vi "gfitsio-error-cluster-from-code.vi"(8 "error in (no error)":errorcluster, 11 "error code":i32) -> (0 "error out":errorcluster)   [LabVIEW 2019, in "gfitsio.lvlib"]
doc: "Converts an error code to an error cluster. If the CFITSIO error stack contains messages, these are placed in the \"source\" field of <B>error out</B>. If <B>error in</B> indicates that an error occurred before this VI or function ran, <B>error out</B> contains the same error information. Otherwise, it describes the error status corresponding to the <B>error code</B>."
uses:
  gfitsio.lvlib
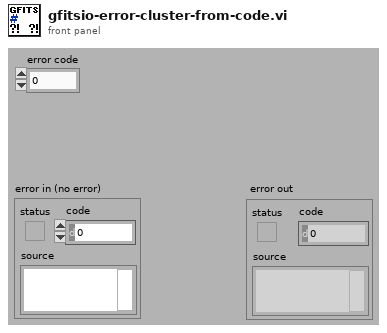
[diagram p1: front panel]
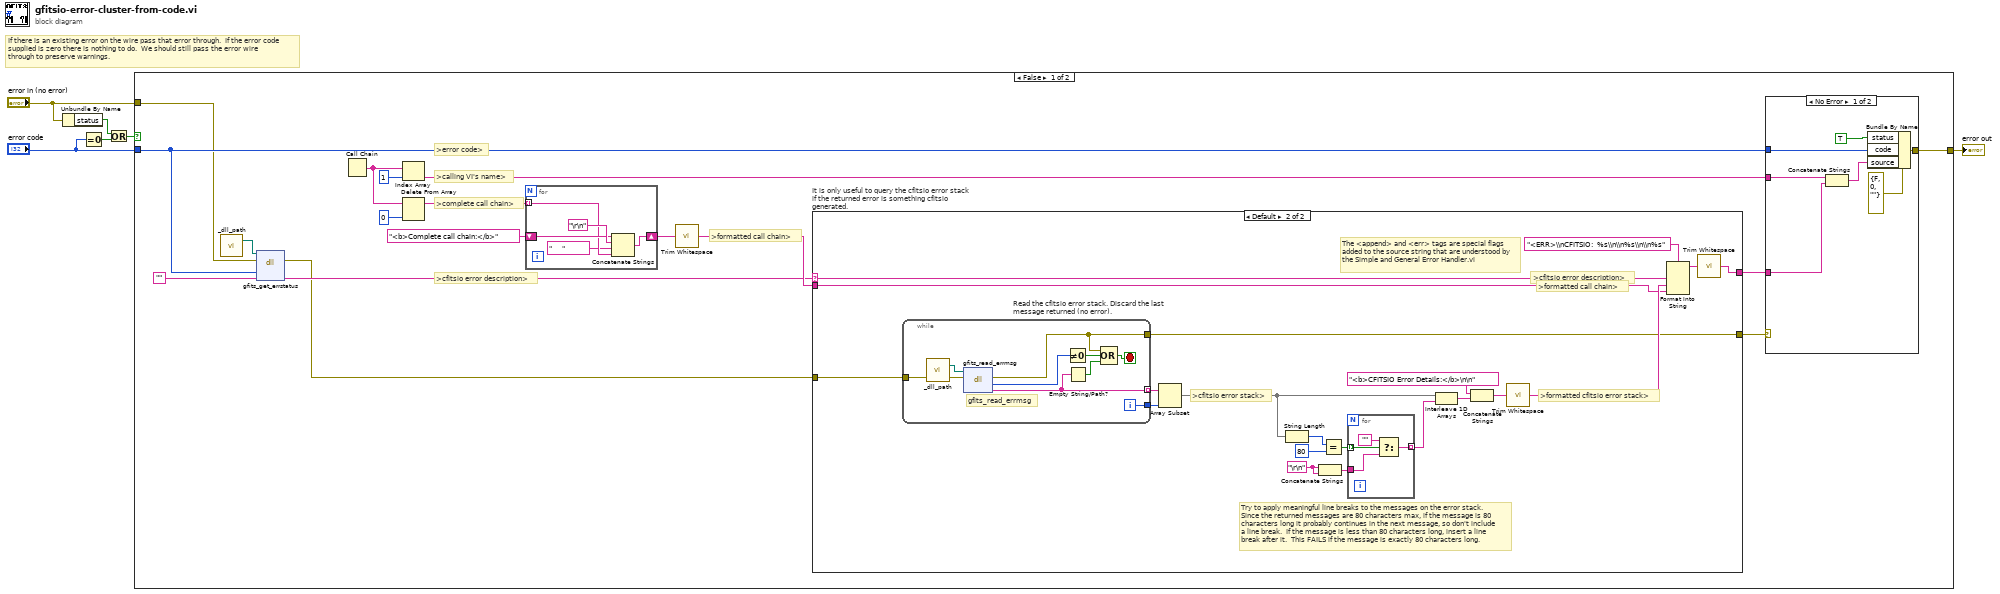
[diagram p0: block diagram]
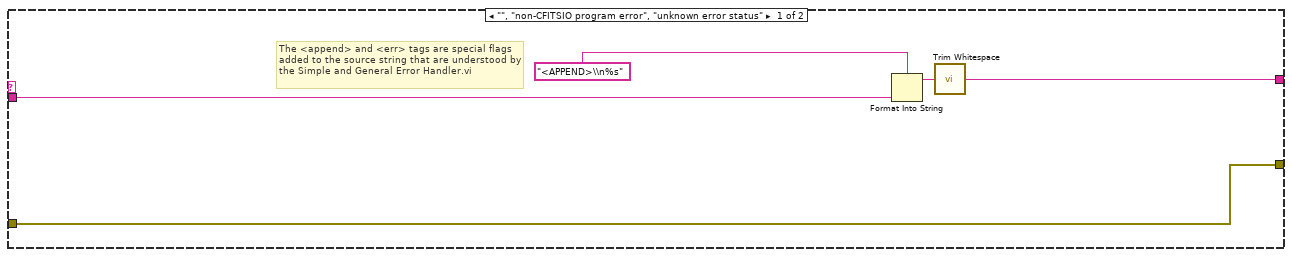
[diagram p3: hidden frame]
diagram:
  # "If there is an existing error on the wire pass that error through.  If the error code supplied is zero there is nothing to do.  We should still pass the error wire through to preserve warnings."
  n1 = Unbundle By Name("error in (no error)") -> ("status"=w4:bool)
  n2 = Equal To 0?(x="error code") -> (x = 0?=w5:bool)
  n3 = Or(x=w4, y=w5) -> (x .or. y?=w3:bool)
  n4 = case shown="False" w3 {
    tunnel: "error code" -> [w12 _]
    tunnel: "error in (no error)" -> [w9 w75]
    tunnel: [w11 w75] -> w1
    frame False {
      # ">formatted call chain>"
      # ">cfitsio error description>"
      # ">complete call chain>"
      # ">calling VI's name>"
      # ">error code>"
      n5 = call "_dll_path.vi"() -> ("Path"=w10:path)  [unwired: 1 in]
      n6 = dll-call lib="?" fn="gfits_get_errstatus"(path in=w10, error in=w9, "status"=w12, "err_text"="") -> (error out=w8:errorcluster, "err_text"=w13:string)  [unwired: 2 in, 2 out]
      n7 = Call Chain() -> (call chain=w20:string[])
      n8 = Index Array(array=w20, index=1) -> (element=w16:string)
      n9 = Delete From Array(array=w20, index=0) -> (array with subset deleted=w22:string[])  [unwired: 1 in, 1 out]
      n10 = for {
        tunnel: w22 -> [w71] mode=indexing
        shift-right: [w74] -> w15
        shift-left: "<b>Complete call chain:</b>" ("call chain header") -> [w72]
        n11 = Concatenate Strings(w72, "\r\n", "     ", w71) -> (w74:string)
      }
      n12 = call <vilib>:"Trim Whitespace.vi"("string"=w15) -> ("trimmed string"=w14:string)  [unwired: 1 in]
      n13 = case "It is only useful to query the cfitsio error stack if the returned error is something cfitsio generated." shown="Default" w13 {
        selector: w13 -> [_ w39]
        tunnel: [w34 w52] -> w17
        tunnel: w14 -> [w33 w40]
        tunnel: w8 -> [w32 w38]
        tunnel: [w32 w37] -> w7
        frame "", "non-CFITSIO program error", "unknown error status" {
          # "The <append> and <err> tags are special flags added to the source string that are understood by the Simple and General Error Handler.vi"
          n14 = Format Into String(format string="<APPEND>\\n%s", w33) -> (resulting string=w36:string)  [unwired: 2 in, 1 out]
          n15 = call <vilib>:"Trim Whitespace.vi"("string"=w36) -> ("trimmed string"=w34:string)  [unwired: 1 in]
        }
        frame Default {
          w45 = "\r\n"
          # ">cfitsio error description>"
          # ">formatted call chain>"
          # "The <append> and <err> tags are special flags added to the source string that are understood by the Simple and General Error Handler.vi"
          # ">formatted cfitsio error stack>"
          # "Try to apply meaningful line breaks to the messages on the error stack.  Since the returned messages are 80 characters max, if the message is 80 characters long it probably continues in the next message, so don't include a line break.  If the message is less than 80 characters long, insert a line break after it.  This FAILS if the message is exactly 80 characters long."
          # ">cfitsio error stack>"
          n16 = while "Read the cfitsio error stack. Discard the last message returned (no error)." {
            tunnel: [w69] -> w56 mode=indexing
            tunnel: [w68] -> w55
            tunnel: w38 -> [w62]
            tunnel: [w61] -> w37
            i -> [w68]
            stop <- w64 stop-if-true
            # "gfits_read_errmsg"
            n17 = call "_dll_path.vi"() -> ("Path"=w63:path)  [unwired: 1 in]
            n18 = dll-call lib="?" fn="gfits_read_errmsg"(path in=w63, error in=w62) -> (error out=w61:errorcluster, "return type"=w67:i32, "err_text"=w69:string)  [unwired: 1 in, 2 out]
            n19 = Not Equal To 0?(x=w67) -> (x != 0?=w65:bool)
            n20 = Empty String/Path?(string/path=w69) -> (empty?=w66:bool)
            n21 = Compound Arithmetic op=OR(w61, w65, w66) -> (w64:bool)
          }
          n22 = Array Subset(array=w56, length=w55) -> (w43:string[])  [unwired: 1 in]
          n23 = String Length(string=w43) -> (length=w50:i32[])
          n24 = Concatenate Strings(w45, w45) -> (w44:string)
          n25 = Equal?(x=w50, y=80) -> (x = y?=w48:bool[])
          n26 = for {
            tunnel: w48 -> [w60] mode=indexing
            tunnel: [w58] -> w47 mode=indexing
            tunnel: w44 -> [w57]
            n27 = Select(t="", s=w60, f=w57) -> (s? t:f=w58:string)
          }
          n28 = Interleave 1D Arrays(w43, w47) -> (w46:string[])
          n29 = Concatenate Strings("<b>CFITSIO Error Details:</b>\n\n" ("string"), w46) -> (w42:string)
          n30 = call <vilib>:"Trim Whitespace.vi"("string"=w42) -> ("trimmed string"=w41:string)  [unwired: 1 in]
          n31 = Format Into String(format string="<ERR>\\nCFITSIO:  %s\\n\\n%s\\n\\n%s", w39, w41, w40) -> (resulting string=w54:string)  [unwired: 2 in, 1 out]
          n32 = call <vilib>:"Trim Whitespace.vi"("string"=w54) -> ("trimmed string"=w52:string)  [unwired: 1 in]
        }
      }
      n33 = case shown="No Error" w7 {
        selector: w7 -> [_ w31]
        tunnel: w17 -> [w27 _]
        tunnel: w16 -> [w26 _]
        tunnel: w12 -> [w25 _]
        tunnel: [w24 w31] -> w11
        frame No Error {
          n34 = Concatenate Strings(w26, w27) -> (w29:string)
          n35 = Bundle By Name(cluster=errorcluster {"status"=FALSE, "code"=0, "source"=""} ("error out"), "status"=TRUE, "code"=w25, "source"=w29) -> (w24:errorcluster)
        }
        frame Error {
        }
      }
    }
    frame True {
    }
  }
  "error out" <- w1
